vi "Check Alias for Reserved Keywords.vi"(6 "Reserved Keywords":string[](array[string])=["All_Photons", "F_D^D", "F_D^_A", "F_A^_D", "F_A^A", "F_D^M", "F_A^M", "Donor", "Acceptor", "FRET", "ALEX", "t_burst", "B_All", "B_D^D", "B_D^A", "B_A^D", "B_A^A", "B^D", "B^A"], 9 "Alias Name":string, 11 "Aliases Array in":string[](array[string])) -> (0 "Keyword":string, 1 "Is Part of Reserved Keywords":bool, 2 "index of element":i32, 3 "Duplicate":bool)   [LabVIEW 2021, in "Formula.lvlib"]
uses:
  Formula.lvlib
  Formula VIs Functions.ctl
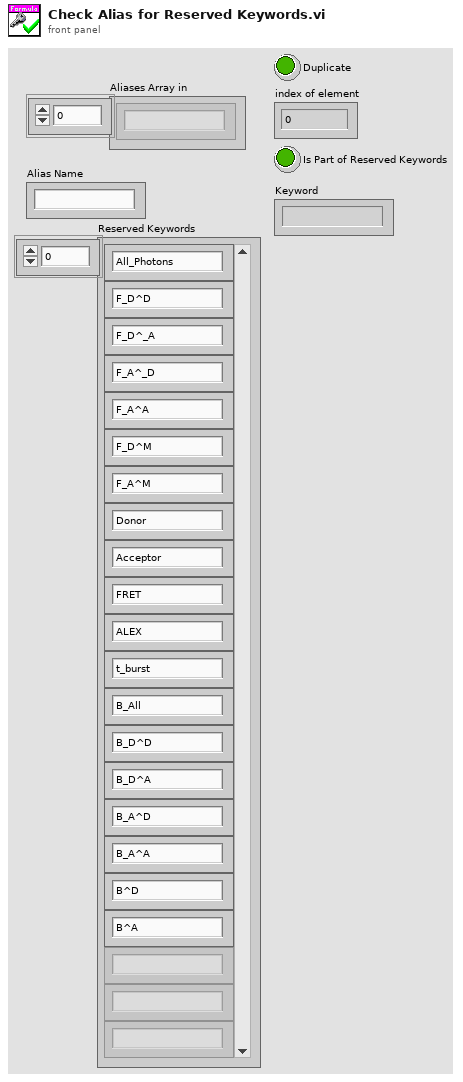
[diagram p1: front panel]
types:
  T1 = typedef "Formula.lvlib/Formula VIs Functions.ctl" = string[]
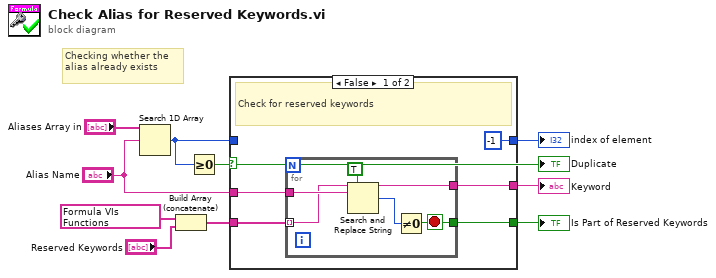
[diagram p0: block diagram]
diagram:
  # "Checking whether the alias already exists"
  n1 = Search 1D Array(1D array="Aliases Array in", element="Alias Name") -> (index of element=w9:i32)  [unwired: 1 in]
  n2 = Build Array (concatenate)(T1 ["abs", "acos", "acosh", "asin", "asinh", "atan", "atanh", "ceil", "cos", "cosh", "cot", "csc", "exp", "expm1", "floor", "getexp", "getman", "int", "intrz", "ln", "lnp1", "log", "log2", "rand", "sec", "sign", "sin", "sinc", "sinh", "sqrt", "tan", "tanh", "gamma", "pi", "ci", "si", "spike", "step", "square"] ("Function Array"), "Reserved Keywords") -> (w3:T1)
  n3 = Greater Or Equal To 0?(x=w9) -> (x >= 0?=w10:bool)
  "Duplicate" <- w10
  n4 = case shown="False" w10 {
    tunnel: w9 -> [_ w21]
    tunnel: [-1 ("index of element") w21] -> w8
    tunnel: [w13 _] -> w7
    tunnel: "Alias Name" -> [w12 _]
    tunnel: w3 -> [w15 _]
    tunnel: [w11 _] -> w1
    frame False {
      # "Check for reserved keywords"
      n5 = for {
        tunnel: w15 -> [w16] mode=indexing
        tunnel: [w19] -> w13
        tunnel: w12 -> [w18]
        tunnel: [w16] -> w11
        stop <- w19 stop-if-true
        n6 = Search and Replace String(replace all?=TRUE ("replace all? (F)"), input string=w16, search string=w18) -> (number of replacements=w20:i32)  [unwired: 5 in, 3 out]
        n7 = Not Equal To 0?(x=w20) -> (x != 0?=w19:bool)
      }
    }
    frame True {
    }
  }
  "index of element" <- w8
  "Is Part of Reserved Keywords" <- w7
  "Keyword" <- w1
